vi "gmail.vi"() -> ()   [LabVIEW 2014]
panel:
  in  "CC (Carbon Copy Recipient - Optional)":string
  in  "Attachment - Optional":path
  in  "Port":i32=587
  in  "Enable SSL":bool=TRUE
  in  "GMAIL Account Password":string
  in  "GMAIL Account User ID (eg: jsmity77)":string
  in  "Outgoing Mail Server (SMTP)":string="smtp.gmail.com"
  in  "Body":string="It works!"
  in  "Subject":string="Sending TLS Authenticated Email"
  in  "Recipient's Name":string="Jane Doe"
  in  "Recipient's Email Address Address":string
  in  "Sender's Name":string="John Smith"
  in  "Sender's Email Address (eg: jsmith77@gmail.com)":string
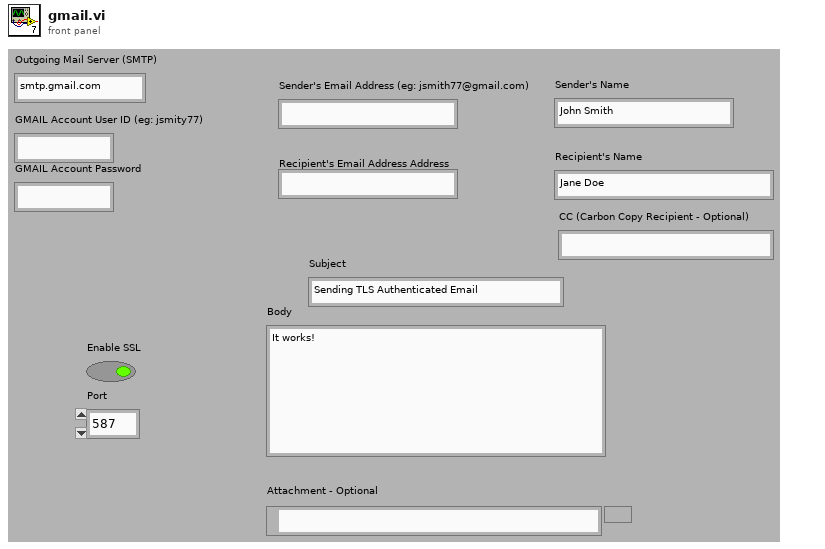
[diagram p1: front panel]
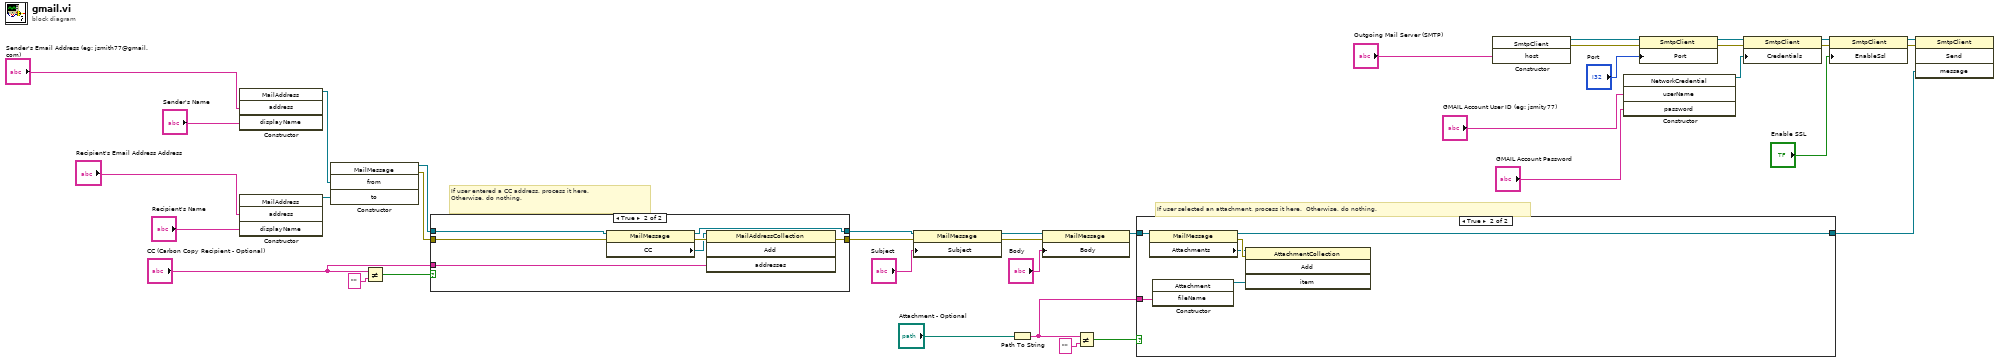
[diagram p0: block diagram]
diagram:
  # "If user selected an attachment, process it here.  Otherwise, do nothing."
  # "If user entered a CC address, process it here.\nOtherwise, do nothing."
  n1 = constructor class="MailAddress"("address"="Sender's Email Address (eg: jsmith77@gmail.com)", "displayName"="Sender's Name") -> (reference out=w36:refnum<k24>)  [unwired: 3 in, 4 out]
  n2 = constructor class="MailAddress"("address"="Recipient's Email Address Address", "displayName"="Recipient's Name") -> (reference out=w37:refnum<k24>)  [unwired: 3 in, 4 out]
  n3 = constructor class="MailMessage"("from"=w36, "to"=w37) -> (reference out=w4:refnum<k24>, error out=w3:errorcluster)  [unwired: 3 in, 3 out]
  n4 = Not Equal?(x="CC (Carbon Copy Recipient - Optional)", y="") -> (x != y?=w6:bool)
  n5 = case shown="True" w6 {
    tunnel: "CC (Carbon Copy Recipient - Optional)" -> [_ w44]
    tunnel: w4 -> [w39 w43]
    tunnel: w3 -> [w38 w42]
    tunnel: [w39 w41] -> w2
    tunnel: [w38 w40] -> w1
    frame False {
    }
    frame True {
      n6 = property class="MailMessage"(reference=w43, error in=w42) -> (reference out=w41:refnum<k24>, error out=w46:errorcluster, "CC"=w45:refnum<k24>)
      n7 = invoke class="MailAddressCollection" method="Add"(reference=w45, error in=w46, "addresses"=w44) -> (error out=w40:errorcluster)  [unwired: 1 in, 3 out]
    }
  }
  n8 = property class="MailMessage"(reference=w2, error in=w1, "Subject"="Subject") -> (reference out=w27:refnum<k24>, error out=w35:errorcluster)
  n9 = Path To String(path="Attachment - Optional") -> (string=w8:string)
  n10 = property class="MailMessage"(reference=w27, error in=w35, "Body"="Body") -> (reference out=w13:refnum<k24>)  [unwired: 1 out]
  n11 = Not Equal?(x=w8, y="") -> (x != y?=w9:bool)
  n12 = case shown="True" w9 {
    tunnel: w13 -> [w47 w50]
    tunnel: [w47 w49] -> w12
    tunnel: w8 -> [_ w48]
    frame False {
    }
    frame True {
      n13 = property class="MailMessage"(reference=w50) -> (reference out=w49:refnum<k24>, error out=w53:errorcluster, "Attachments"=w51:refnum<k24>)  [unwired: 1 in]
      n14 = constructor class="Attachment"("fileName"=w48) -> (reference out=w52:refnum<k24>)  [unwired: 3 in, 3 out]
      n15 = invoke class="AttachmentCollection" method="Add"(reference=w51, error in=w53, "item"=w52) -> ()  [unwired: 1 in, 4 out]
    }
  }
  n16 = constructor class="SmtpClient"("host"="Outgoing Mail Server (SMTP)") -> (reference out=w21:refnum<k24>, error out=w17:errorcluster)  [unwired: 3 in, 2 out]
  n17 = constructor class="NetworkCredential"("userName"="GMAIL Account User ID (eg: jsmity77)", "password"="GMAIL Account Password") -> (reference out=w22:refnum<k24>)  [unwired: 3 in, 4 out]
  n18 = property class="SmtpClient"(reference=w21, error in=w17, "Port"="Port") -> (reference out=w20:refnum<k24>, error out=w16:errorcluster)
  n19 = property class="SmtpClient"(reference=w20, error in=w16, "Credentials"=w22) -> (reference out=w19:refnum<k24>, error out=w15:errorcluster)
  n20 = property class="SmtpClient"(reference=w19, error in=w15, "EnableSsl"="Enable SSL") -> (reference out=w18:refnum<k24>, error out=w14:errorcluster)
  n21 = invoke class="SmtpClient" method="Send"(reference=w18, error in=w14, "message"=w12) -> ()  [unwired: 1 in, 4 out]
